vi "Interpolate IQ (8spc).vi"(0 "data in FIFO":refnum<k21>, 1 "Clock x2":refnum<k21>, 5 "data out FIFO - interpolated":refnum<k21>, 7 "input sample rate":fxp<+,48,1>, 12 "burst size":u32, 14 "reset":bool) -> (4 "count out":u32, 6 "input consumed":bool[](array[boolean]))   [LabVIEW 2019]
uses:
  16 spc U32 array.ctl
  <instrlib>/_niInstr/DSP/v1/Shared/Public/IQ Data.ctl
  <vilib>/rvi/DataTransferAndStorage/Container/Common/niFpgaContainerExecOnDevCompGetState.vi
  <vilib>/rvi/Emulation/niFpgaSctlEmulationGetInTimedLoop.vi
  <vilib>/rvi/errors/niFpgaSetErrorForExecOnDevCompSimple.vi
  <vilib>/rvi/eio/common/nirviEmuReportErrorAndStop.vi
  <vilib>/rvi/interface/RandomDataEmulation/nirviRandomDataAcquireLock.vi
  <vilib>/rvi/interface/RandomDataEmulation/nirviRandomDataQueueStore.vi
  <vilib>/rvi/interface/RandomDataEmulation/nirviRandomDataReleaseLock.vi
  <vilib>/rvi/interface/RandomDataEmulation/nirviFPGAContextMergeError.vi
  <vilib>/rvi/interface/RandomDataEmulation/nirviRandomDataCheckExitLoopConditions.vi
  <vilib>/express/rvi/timingcommon/nirviCommon.vi
  <vilib>/rvi/interface/RandomDataEmulation/niFpgaRandomDataHandleErrors.vi
  <instrlib>/_niInstr/Basic Elements/v1/FPGA/Private/Count Up U32.vi
  <instrlib>/_niInstr/DSP/v1/FPGA/Public/Sub VIs/Fractional Interpolator/Fractional Interpolator - 8 spc - 2x oc.vi
  <vilib>/rvi/Emulation/niFpgaEmulationIsFPGAContextNoSignature.vi
  <vilib>/rvi/DataTransferAndStorage/Container/Common/niFpgaContainerGetUniqueNameForEmu.vi
  <vilib>/rvi/FIFO/Fifo_Resource/nirvififoEmulationSetSize.vi
  <vilib>/rvi/FIFO/Fifo_Resource/nirviFifoEmulationQueueMgr.vi
  <instcachedir>/0/nirviFifoEmulationQueueMgr_E5CAEC123FF24DC58D834DCA3CDAA9B5.lvgen/nirviFifoEmulationQueueMgr_E5CAEC123FF24DC58D834DCA3CDAA9B5_008.vi
  <vilib>/rvi/FIFO/Fifo_Resource/nirvififoEmulationDetermineInputValidOut.vi
  <vilib>/rvi/FIFO/Fifo_Resource/nirvififoEmulationCreateLock.vi
  <vilib>/rvi/Emulation/niFpgaProcessEmulError.vi
  <vilib>/rvi/FIFO/Fifo_Resource/nirvififoEmulationObtainLock.vi
  <vilib>/rvi/FIFO/Fifo_Resource/nirvififoEmulationReleaseLock.vi
  <vilib>/rvi/occurrence/nirviWaitOnOccurrenceBase.vi
  <vilib>/rvi/errors/nirviReportUnexpectedCaseInternalError.vi
  <vilib>/rvi/errors/nirviReportUnexpectedCaseInternalError (U32).vi
  <vilib>/Utility/error.llb/Clear Errors.vi
  <vilib>/rvi/DataTransferAndStorage/Container/XNode/niFpgaContainer.xnode
  <vilib>/rvi/FIFO/Fifo_Resource/niFpgaFifoEmulationRefInMultiElement.vi
  <vilib>/rvi/FIFO/Fifo_Resource/niFpgaFifoEmulationRefIn.vi
  <instrlib>/_niInstr/DSP/v1/Shared/niInstr DSP v1 Shared.lvlib
  <instrlib>/_niInstr/DSP/v1/FPGA/niInstr DSP v1 FPGA.lvlib
  <instrlib>/_niInstr/Basic Elements/v1/FPGA/niInstr Basic Elements v1 FPGA.lvlib
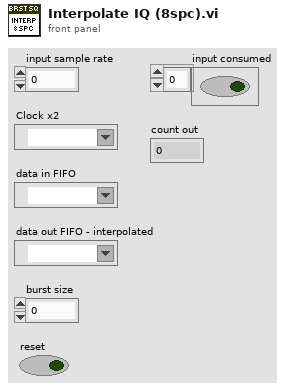
[diagram p1: front panel]
types:
  T1 = typedef "16 spc U32 array.ctl" = u32[]
  T2 = typedef "niInstr DSP v1 Shared.lvlib/IQ Data.ctl" = cluster{"I":fxp<+/-,18,1>, "Q":fxp<+/-,18,1>, "overflow":bool}
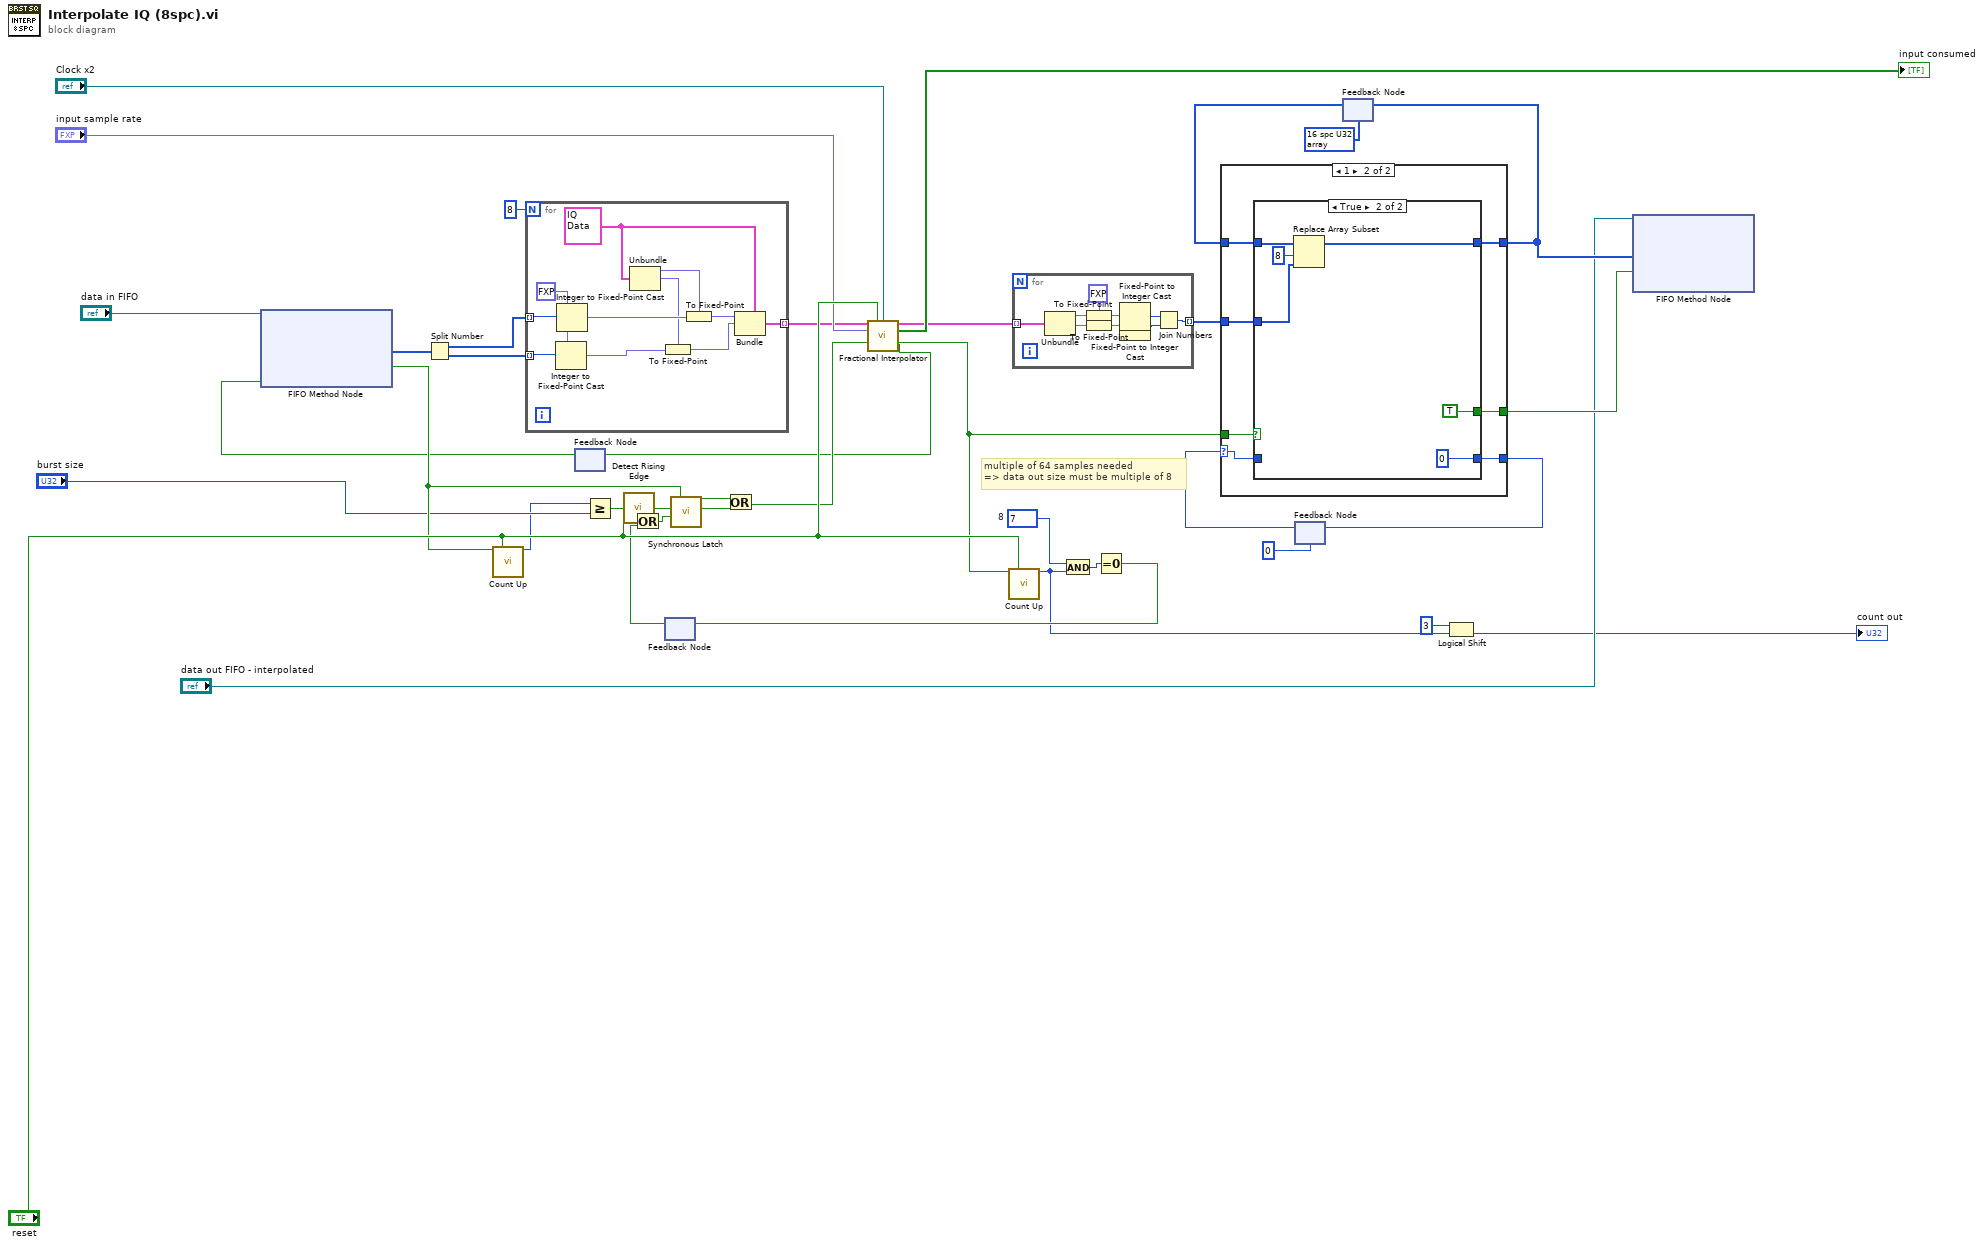
[diagram p0: block diagram]
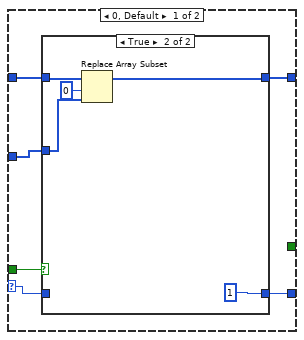
[diagram p2: hidden frame]
diagram:
  w29 = u32 7  # 8
  # "multiple of 64 samples needed\n=> data out size must be multiple of 8"
  n1 = feedback #1() -> (w1:bool)  [unwired: 1 in]
  n2 = xnode ("FIFO Method Node")("Ready for Output"=w1, "FIFO In"="data in FIFO") -> ("Element"=w6:u32[], "Output Valid"=w35:bool)  [unwired: 1 out]
  n3 = Split Number(x=w6) -> (hi(x)=w7:u16[], lo(x)=w8:u16[])
  n4 = call-poly <instrlib>:"Count Up.vi"("increment"=w35, "reset"="reset") -> ("count out"=w24:u32)  [unwired: 13 in]
  n5 = for {
    N: 8 -> [_]
    tunnel: w7 -> [w49] mode=indexing
    tunnel: w8 -> [w48] mode=indexing
    tunnel: [w39] -> w11 mode=indexing
    w40 = T2 {"I"=0.0, "Q"=0.0, "overflow"=FALSE} ("data")
    w47 = fxp<+/-,16,1> 0.0 ("fixed-point type")
    n6 = Integer to Fixed-Point Cast(fixed-point type=w47, integer=w48) -> (fixed-point=w45:fxp<+/-,16,1>)
    n7 = Integer to Fixed-Point Cast(fixed-point type=w47, integer=w49) -> (fixed-point=w46:fxp<+/-,16,1>)
    n8 = Unbundle(w40) -> ("I"=w44:fxp<+/-,18,1>, "Q"=w43:fxp<+/-,18,1>)  [unwired: 1 out]
    n9 = To Fixed-Point(fixed-point type=w43, number=w45) -> (fixed-point=w41:fxp<+/-,18,1>)
    n10 = To Fixed-Point(fixed-point type=w44, number=w46) -> (fixed-point=w42:fxp<+/-,18,1>)
    n11 = Bundle(cluster=w40, "I"=w42, "Q"=w41) -> (w39:T2)  [unwired: 1 in]
  }
  n12 = Greater Or Equal?(x=w24, y="burst size") -> (x >= y?=w32:bool)
  n13 = call <instrlib>:"Detect Rising Edge.vi"("signal"=w32) -> ("edge detected"=w3:bool)  [unwired: 14 in]
  n14 = feedback #2() -> (w33:bool)  [unwired: 1 in]
  n15 = Or(x="reset", y=w33) -> (x .or. y?=w37:bool)
  n16 = call <instrlib>:"Synchronous Latch.vi"("clear"=w37, "set"=w3) -> ("out"=w34:bool)  [unwired: 9 in]
  n17 = Or(x=w35, y=w34) -> (x .or. y?=w36:bool)
  n18 = call-poly <instrlib>:"Fractional Interpolator.vi"("data in"=w11, "reset"="reset", "clock x 2"="Clock x2", "input sample rate"="input sample rate", "input valid"=w36) -> ("data out"=w12:T2[], "input consumed"=→"input consumed":bool[], "output valid"=w27:bool, "ready for input"=w2:bool)  [unwired: 7 in]
  n19 = feedback-in #1(w2) -> ()
  n20 = call-poly <instrlib>:"Count Up.vi"("increment"=w27, "reset"="reset") -> ("count out"=w28:u32)  [unwired: 13 in]
  n21 = for {
    tunnel: w12 -> [w58] mode=indexing
    tunnel: [w50] -> w19 mode=indexing
    w56 = fxp<+/-,16,1> 0.0 ("fixed-point type")
    n22 = Unbundle(w58) -> ("I"=w57:fxp<+/-,18,1>, "Q"=w55:fxp<+/-,18,1>)  [unwired: 1 out]
    n23 = To Fixed-Point(fixed-point type=w56, number=w57) -> (fixed-point=w54:fxp<+/-,16,1>)
    n24 = To Fixed-Point(fixed-point type=w56, number=w55) -> (fixed-point=w53:fxp<+/-,16,1>)
    n25 = Fixed-Point to Integer Cast(1:w54) -> (0:w52:i16)
    n26 = Fixed-Point to Integer Cast(1:w53) -> (0:w51:i16)
    n27 = Join Numbers(hi=w52, lo=w51) -> ((hi.lo)=w50:u32)
  }
  n28 = And(x=w29, y=w28) -> (x .and. y?=w30:u32)
  n29 = Equal To 0?(x=w30) -> (x = 0?=w31:bool)
  n30 = feedback-in #2(w31) -> ()
  n31 = feedback #3(i8 0) -> (w15:i8)
  n32 = feedback #4(T1 [0, 0, 0, 0, 0, 0, 0, 0, 0, 0, 0, 0, 0, 0, 0, 0]) -> (w17:T1)
  n33 = case shown="1" w15 {
    selector: w15 -> [w59 w73]
    tunnel: w27 -> [w60 w74]
    tunnel: w17 -> [w63 w77]
    tunnel: [w64 w78] -> w22
    tunnel: w19 -> [w62 w76]
    tunnel: [w61 w75] -> w18
    tunnel: [_ w72] -> w21
    frame 0, Default {
      n34 = case shown="True" w60 {
        tunnel: [w66 w67] -> w64
        tunnel: w63 -> [w66 w71]
        tunnel: w62 -> [_ w70]
        tunnel: [w65 i8 1] -> w61
        tunnel: w59 -> [w65 _]
        frame False {
        }
        frame True {
          n35 = Replace Array Subset(array=w71, new element=w70, index=0) -> (w67:T1)
        }
      }
    }
    frame 1 {
      n36 = case shown="True" w74 {
        tunnel: [w80 w81] -> w78
        tunnel: w77 -> [w80 w86]
        tunnel: w76 -> [_ w85]
        tunnel: [w79 i8 0] -> w75
        tunnel: w73 -> [w79 _]
        tunnel: [_ TRUE] -> w72
        frame False {
        }
        frame True {
          n37 = Replace Array Subset(array=w86, new element=w85, index=8) -> (w81:T1)
        }
      }
    }
  }
  n38 = feedback-in #3(w18) -> ()
  n39 = feedback-in #4(w22) -> ()
  n40 = Logical Shift(y=i16 3, x=w28) -> (x << y=→"count out":u32)
  n41 = xnode ("FIFO Method Node")("Element"=w22, "Input Valid"=w21, "FIFO In"="data out FIFO - interpolated") -> ()  [unwired: 2 out]
